vi "Create Trigger Channel.vi"(8 "error in (no error)":errorcluster, 10 "Channel Parameters":T2, 11 "Message Channels Section in":T1 format="%.0x") -> (0 "error out":errorcluster, 2 "Channel Ref":T1 format="%.0x", 3 "Message Channels Section out":T1 format="%.0x")   [LabVIEW 2020, in "Instrument Addon Scripting API.lvlib"]
uses:
  Instrument Addon Scripting API.lvlib
  <vilib>/NI VeriStand/Custom Device API/Custom Device Item Ref.ctl
  <vilib>/NI VeriStand/Custom Device API/Custom Device Channel.ctl
  <vilib>/NI VeriStand/Custom Device API/Custom Device Channel Type.ctl
  Addon/Addon Shared/SubVIs/Constants.vi
  Addon/Addon Shared/Instrument Addon Shared.lvlib
  <vilib>/NI VeriStand/Custom Device API/Custom Device API.lvlib
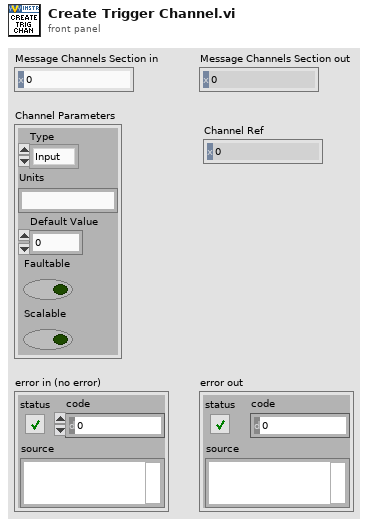
[diagram p1: front panel]
types:
  T1 = typedef "Custom Device API.lvlib/Custom Device Item Ref.ctl" = u64
  T2 = typedef "Custom Device API.lvlib/Custom Device Channel.ctl" = cluster{"Type":T3, "Units":string, "Default Value":dbl, "Faultable":bool, "Scalable":bool}
  T3 = typedef "Custom Device API.lvlib/Custom Device Channel Type.ctl" = enum16{"Input", "Output"}
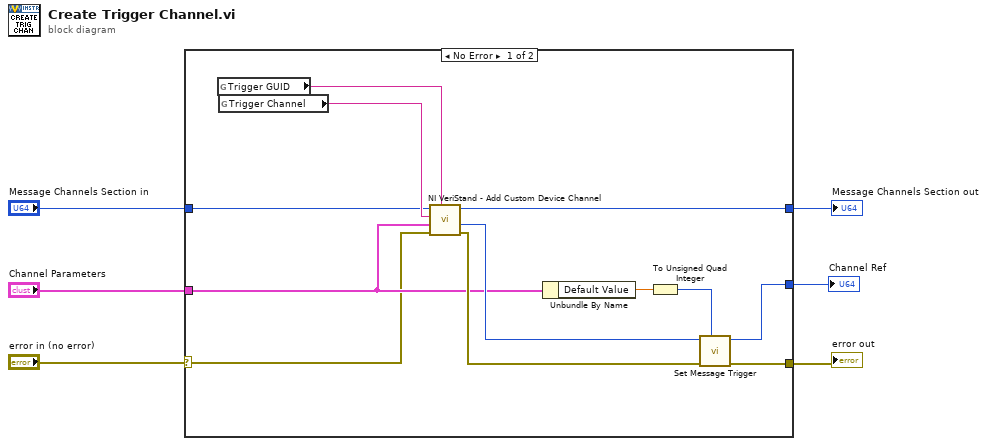
[diagram p0: block diagram]
diagram:
  n1 = case shown="No Error" "error in (no error)" {
    selector: "error in (no error)" -> [w7 w20]
    tunnel: [w18 w19] -> w6
    tunnel: "Message Channels Section in" -> [w15 w19]
    tunnel: [w12 w20] -> w4
    tunnel: [w11 _] -> w3
    tunnel: "Channel Parameters" -> [w10 _]
    frame No Error {
      n2 = global read "Constants.vi" "Trigger GUID"() -> (w16:string)
      n3 = global read "Constants.vi" "Trigger Channel"() -> (w17:string)
      n4 = call <vilib>:"NI VeriStand - Add Custom Device Channel.vi"("GUID (Default Channel)"=w16, "error in (no error)"=w7, "Channel"=w10, "Channel Name"=w17, "Parent Ref in"=w15) -> ("error out"=w14:errorcluster, "Channel Ref"=w13:T1, "Parent Ref out"=w18:T1)  [unwired: 3 in, 1 out]
      n5 = Unbundle By Name(w10) -> ("Default Value"=w9:dbl)
      n6 = To Unsigned Quad Integer(1:w9) -> (0:w8:u64)
      n7 = call "Set Message Trigger.vi"("nodeID"=w8, "error in (no error)"=w14, "Trigger Channel in"=w13) -> ("error out"=w12:errorcluster, "Trigger Channel out"=w11:T1)  [unwired: 7 in]
    }
    frame Error {
    }
  }
  "Message Channels Section out" <- w6
  "error out" <- w4
  "Channel Ref" <- w3
